vi "Test Draw Something.vi"(8 "error in (no error)":errorcluster, 11 "Test Case In":refnum<class "Game Board Test.lvclass">) -> (0 "error out":errorcluster, 3 "Test Case Out":refnum<class "Game Board Test.lvclass">)   [LabVIEW 2020, in "Game Board Test.lvclass"]
uses:
  Game Board Test.lvclass
  Game Board Test.lvclass/Game Board Test.ctl
  source/Game Board/Game Board.lvclass
  source/Particle.lvclass
  source/Particle/Position.ctl
  b5ae9e31-5043-4f8e-b739-63e401381e9f.vi
  C:/git/astemes-snake-game/source/Particle.lvclass
  C:/git/astemes-snake-game/source/Drawable/Drawable.lvclass
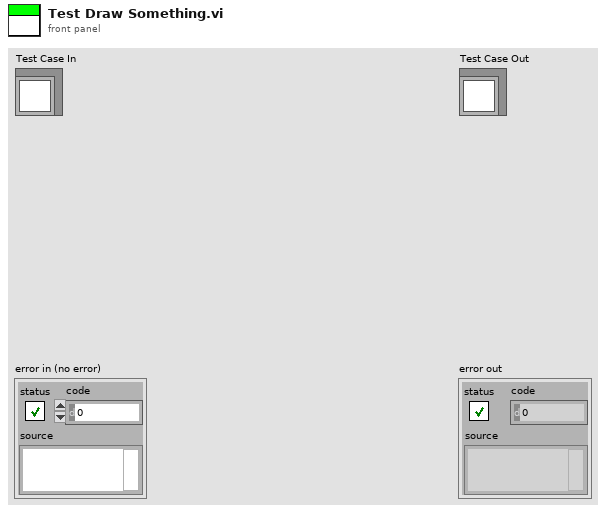
[diagram p1: front panel]
types:
  T1 = typedef "Particle.lvclass/Position.ctl" = cluster{"X":i32, "Y":i32}
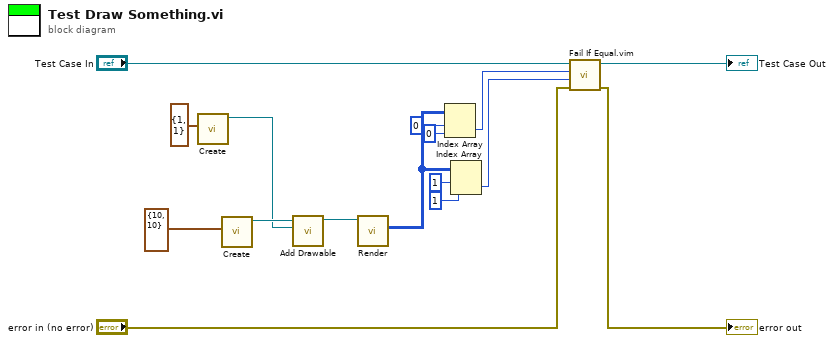
[diagram p0: block diagram]
diagram:
  n1 = call "Create.vi"("Position"=T1 {"X"=1, "Y"=1}) -> ("Particle out"=w9:refnum<class "Particle.lvclass">)  [unwired: 10 in]
  n2 = call "Create.vi"("Size"=cluster{"X":i32, "Y":i32} {"X"=10, "Y"=10}) -> ("Game Board out"=w11:refnum<class "Game Board.lvclass">)  [unwired: 10 in]
  n3 = call "Add Drawable.vi"("Drawable"=w9, "Game Board in"=w11) -> ("Game Board out"=w8:refnum<class "Game Board.lvclass">)  [unwired: 9 in]
  n4 = call "Render.vi"("Game Board in"=w8) -> ("game Board"=w4:u32[][])  [unwired: 9 in, 1 out]
  n5 = Index Array(array=w4, index (row)=0 ("disabled index (row)"), index (col)=0 ("disabled index (col)")) -> (element=w1:u32)
  n6 = Index Array(array=w4, index (row)=1, index (col)=1 ("disabled index (col)")) -> (element=w5:u32)
  n7 = call "Fail If Equal.vim"("error in (no error)"="error in (no error)", "Actual"=w5, "Expected"=w1, "LUnit Test Case In"="Test Case In") -> ("error out"=→"error out":errorcluster, "LUnit Test Case Out"=→"Test Case Out":refnum<class "Game Board Test.lvclass">)  [unwired: 6 in]
